vi "平台远程升级固件.vi"(8 "error in (no error)":errorcluster, 11 "固件升级":enum16{"无", "CODMn", "氨氮", "总磷", "总氮", "CODCr"}(ring)) -> (0 "error out":errorcluster)   [LabVIEW 2016, in "数据传输系统.lvlib" / "update.lvlib" / "http client.lvclass"]
uses:
  http client.lvclass
  update.lvlib
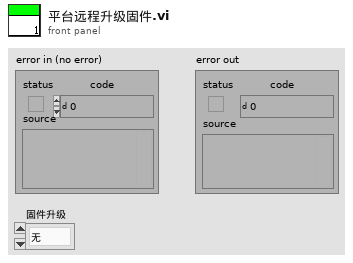
[diagram p1: front panel]
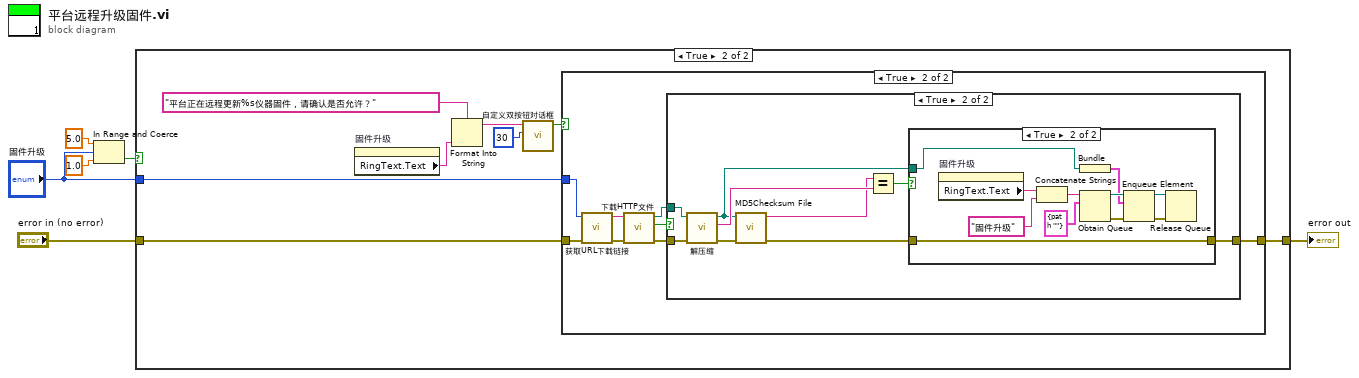
[diagram p0: block diagram]
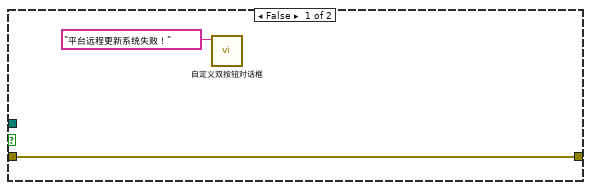
[diagram p4: hidden frame]
diagram:
  n1 = In Range and Coerce(upper limit=5.0 ("上限"), x="固件升级", lower limit=1.0 ("下限")) -> (In Range?=w1:bool)  [unwired: 1 out]
  n2 = case shown="True" w1 {
    tunnel: "error in (no error)" -> [w7 w13]
    tunnel: [w7 w12] -> w5
    tunnel: "固件升级" -> [_ w8]
    frame False {
    }
    frame True {
      n3 = property on="固件升级" class="Enum (严格)"() -> ("RingText.Text"=w10:string)  [unwired: 2 in, 2 out]
      n4 = Format Into String(format string="平台正在远程更新%s仪器固件，请确认是否允许？" ("消息"), w10) -> (resulting string=w9:string)  [unwired: 2 in, 1 out]
      n5 = call "自定义双按钮对话框.vi"("数值"=30, "消息"=w9) -> ("输出"=w14:bool)  [unwired: 9 in]
      n6 = case shown="True" w14 {
        tunnel: w13 -> [w16 w19]
        tunnel: [w16 w18] -> w12
        tunnel: w8 -> [_ w17]
        frame False {
        }
        frame True {
          n7 = call "获取URL下载链接.vi"("error in (no error)"=w19, "固件升级"=w17) -> ("error out"=w22:errorcluster, "String/Binary data"=w21:string)  [unwired: 8 in]
          n8 = call "下载HTTP文件.vi"("error in (no error)"=w22, "Base URL"=w21) -> ("error out"=w23:errorcluster, "ok?"=w20:bool, "路径"=w24:path)  [unwired: 7 in]
          n9 = case shown="True" w20 {
            tunnel: w24 -> [_ w35]
            tunnel: w23 -> [w25 w34]
            tunnel: [w25 w27] -> w18
            frame False {
              n10 = call "自定义双按钮对话框.vi"("消息"="平台远程更新系统失败！") -> ()  [unwired: 10 in, 1 out]
            }
            frame True {
              n11 = call "解压缩.vi"("error in (no error)"=w34, "Zip file"=w35) -> ("error out"=w31:errorcluster, "MD5"=w33:string, "待校验的文件路径"=w30:path)  [unwired: 7 in]
              n12 = call <vilib>:"MD5Checksum File.vi"("error in (no error)"=w31, "Path"=w30) -> ("error out"=w29:errorcluster, "MD5 message-digest"=w32:string)  [unwired: 8 in]
              n13 = Equal?(x=w32, y=w33) -> (x = y?=w28:bool)
              n14 = case shown="True" w28 {
                tunnel: w30 -> [_ w40]
                tunnel: w29 -> [w36 w47]
                tunnel: [w36 w47] -> w27
                frame False {
                }
                frame True {
                  n15 = property on="固件升级" class="Enum (严格)"() -> ("RingText.Text"=w46:string)  [unwired: 2 in, 2 out]
                  n16 = Concatenate Strings(w46, "固件升级" ("字符串")) -> (w43:string)
                  n17 = Bundle("待校验的文件路径"=w40) -> (w39:cluster{"待校验的文件路径":path})  [unwired: 1 in]
                  n18 = Obtain Queue(name (unnamed)=w43, element data type=cluster{"selected path":path} {"selected path"=path ""}) -> (queue out=w42:refnum<queue>, error out=w41:errorcluster)  [unwired: 3 in, 1 out]
                  n19 = Enqueue Element(queue=w42, element=w39, error in (no error)=w41) -> (queue out=w38:refnum<queue>, error out=w37:errorcluster)  [unwired: 1 in, 1 out]
                  n20 = Release Queue(queue=w38, error in (no error)=w37) -> ()  [unwired: 1 in, 3 out]
                }
              }
            }
          }
        }
      }
    }
  }
  "error out" <- w5
